vi "Pockels-Modulate funct acq AO seq for mov cor.vi"(7 "Number of POI":i32=3, 11 "Pockels modulation sequence in":dbl[](array[numeric])=array[5601 elements]) -> (1 "Number of blue block insertions":i32, 3 "Pockels modulation sequence out":dbl[](array[numeric]))   [LabVIEW 2020]
uses:
  Typedefs/Imaging Protocols enum.ctl
  Typedefs/Pockels modulation Internal cluster 1.ctl
  Typedefs/Rounding type.ctl
  Global Variables/General Globals.vi
  Globals/gl_Pockels control globals.vi
panel:
  out "Number of ref frame insertions":i32
  out "Case executing":T1(ring)
  in  "Prevent small final chunks (T)":bool
  out "Size of last chunk as % of nominal chunk size":dbl(slide) scale=0.0..100.0
  in  "Enable simulation slider":bool
  out "Output sequence length (ms)":dbl format="%#_g ms"
  out "Points in o/p sequence":i32 format="%.0f points"
  out "Target time between mov.cor. ref triggers (ms)":dbl=2.0 format="%#_g ms"
  out "Ref frame sequence length (ms)":dbl format="%#_g ms"
  out "nominal chunk length (ms)":dbl format="%#_g ms"
  out "Output Sequence Graph":dbl[](graph)
  in  "Ref frame Pockels modulation sequence size":i32(slide)=376 scale=10.0..1200.0
  out "Insertion indexes":i32[](array[numeric])
  out "Length of pockels mod. seq\nduring ROI acquisition (ms)":dbl=198.0 format="%#_g us"
  # "SIMULATION CONTROL"
  # "<--- This is the total length of the retriggerable sequence shown in the graph"
  # "Output Sequence"
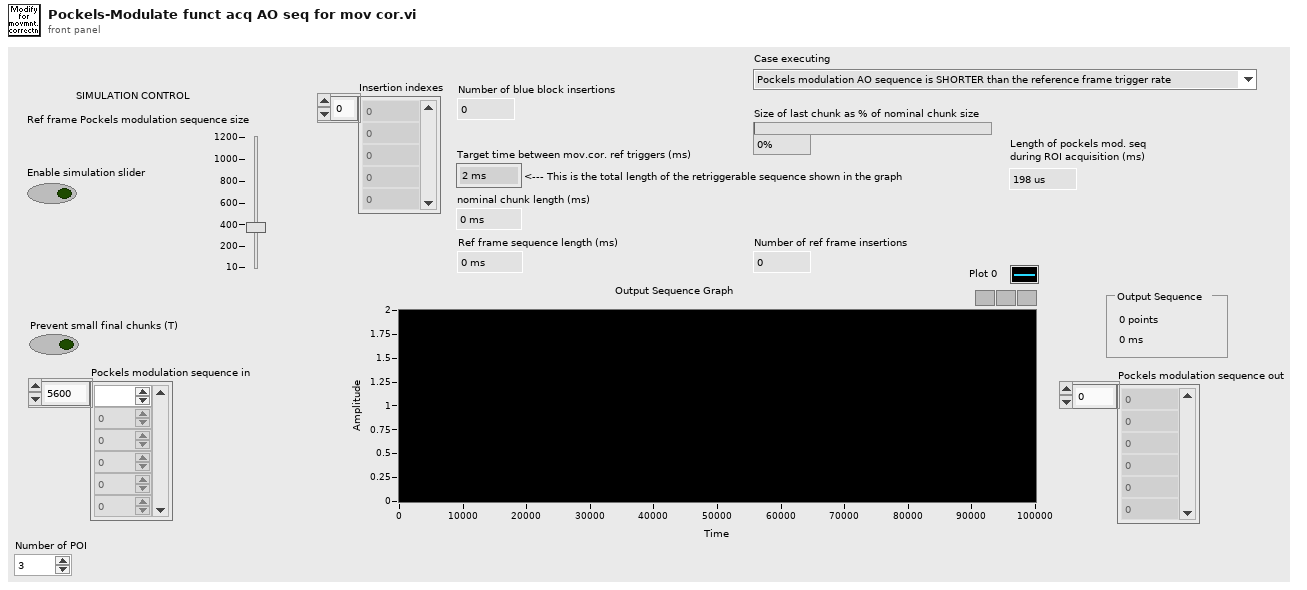
[diagram p1: front panel]
types:
  T1 = enum16{"Pockels modulation AO sequence is SHORTER than the reference frame trigger rate", "Pockels modulation AO sequence is LONGER than the reference frame trigger rate"}
  T2 = typedef "Pockels modulation Internal cluster 1.ctl" = cluster{"Pockels ON \"Pre\" (samples)":i32, "Direction (+-Inf)":T3, "Additional duration to stay ON (samples)":i32, "Not the last ROI":bool}
  T3 = typedef "Rounding type.ctl" = enum16{"No rounding", "Toward +Inf", "Toward -Inf"}
  T4 = typedef "Imaging Protocols enum.ctl" = enum16{"AOL Z-Stack", "Motor Z Stack", "Functional Acquisition", "Single Plane Acquisition", "Volume Acquisition", "Live Imaging", "Live Plane Imaging", "Live Volume Imaging"}
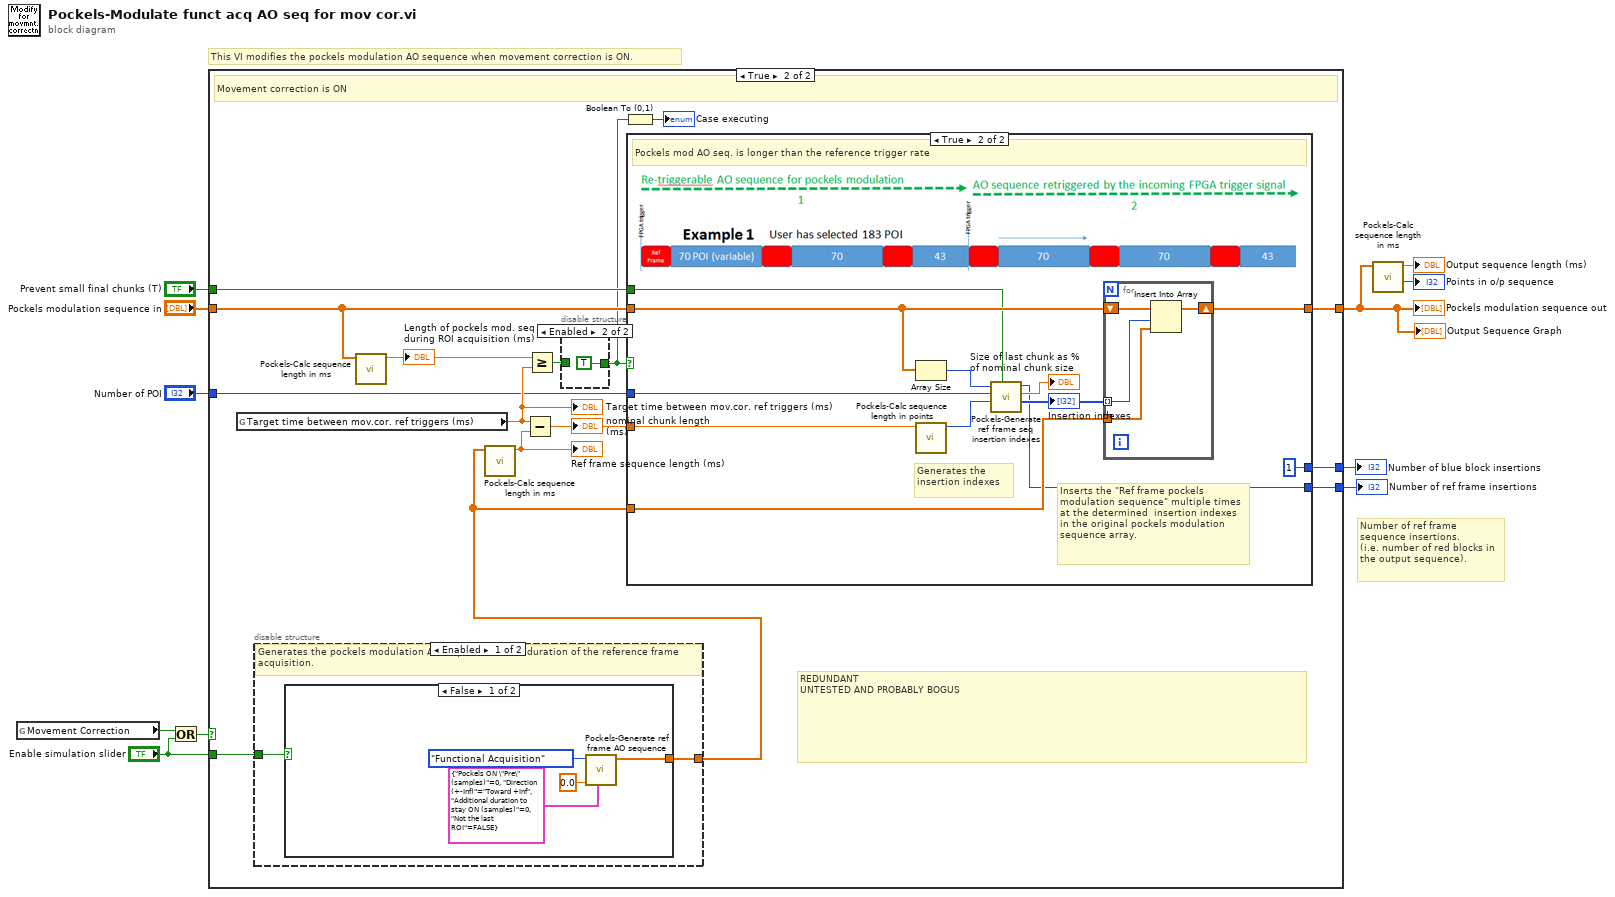
[diagram p0: block diagram]
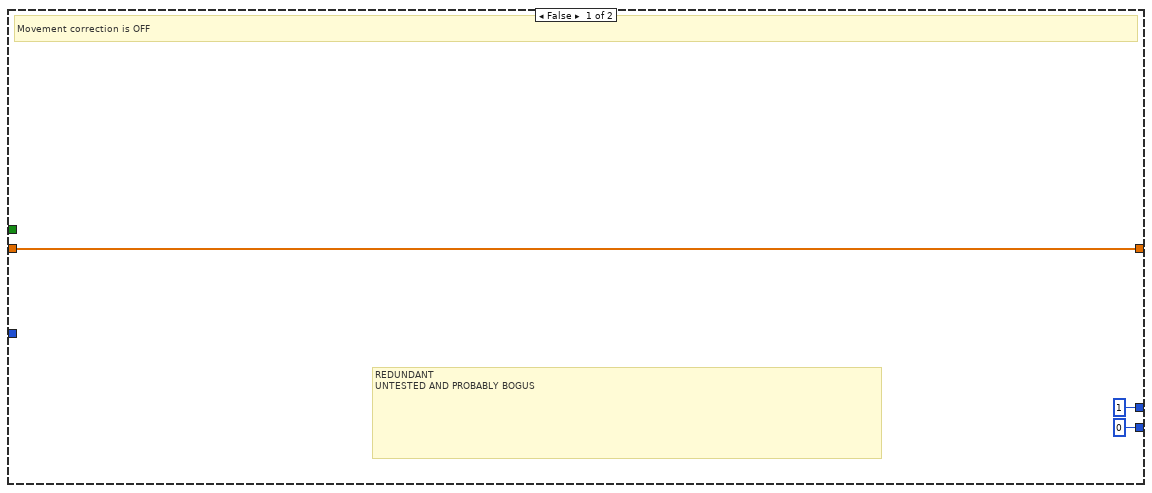
[diagram p2: hidden frame]
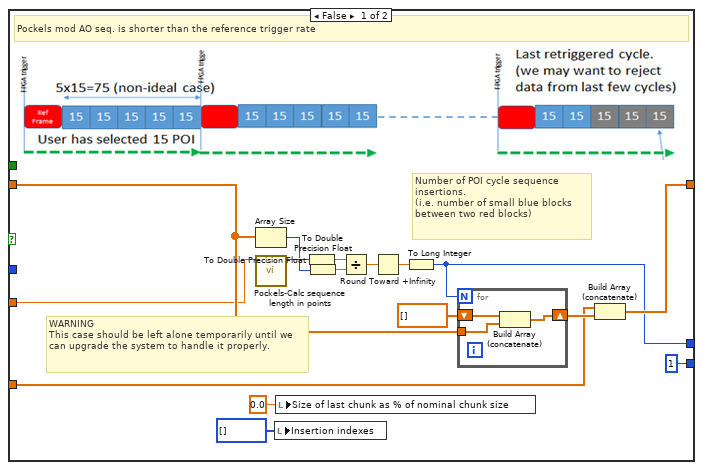
[diagram p4: hidden frame]
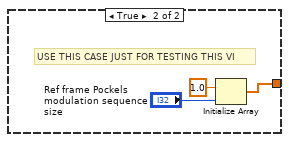
[diagram p5: hidden frame]
diagram:
  # "Number of ref frame sequence insertions.\n(i.e. number of red blocks in the output sequence)."
  # "This VI modifies the pockels modulation AO sequence when movement correction is ON."
  n1 = global read "General Globals.vi" "Movement Correction"() -> (w7:bool)
  n2 = Or(x=w7, y="Enable simulation slider") -> (x .or. y?=w6:bool)
  n3 = case shown="True" w6 {
    tunnel: "Pockels modulation sequence in" -> [w14 w18]
    tunnel: [w14 w28] -> w10
    tunnel: "Enable simulation slider" -> [_ w27]
    tunnel: "Prevent small final chunks (T)" -> [_ w26]
    tunnel: [1 w21] -> w4
    tunnel: [0 ("Number of insertions") w20] -> w3
    tunnel: "Number of POI" -> [_ w17]
    frame False {
      # "REDUNDANT\nUNTESTED AND PROBABLY BOGUS"
      # "Movement correction is OFF"
    }
    frame True {
      # "REDUNDANT\nUNTESTED AND PROBABLY BOGUS"
      # "Movement correction is ON"
      n4 = global read "gl_Pockels control globals.vi" "Target time between mov.cor. ref triggers (ms)"() -> (w22:dbl)
      "Target time between mov.cor. ref triggers (ms)" <- w22
      n5 = disable-structure shown="Enabled" {
        disable-tunnel: [w68 _] -> w19
        disable-tunnel: w27 -> [w67 _]
        frame Enabled {
          # "Generates the pockels modulation AO sequence for the duration of the reference frame acquisition."
          n6 = case shown="False" w67 {
            tunnel: [w72 w73] -> w68
            frame False {
              n7 = call "Pockels-Generate ref frame AO sequence.vi"("Cluster"=T2 {"Pockels ON \"Pre\" (samples)"=0, "Direction (+-Inf)"=enum."Toward +Inf", "Additional duration to stay ON (samples)"=0, "Not the last ROI"=FALSE}, "Previous excess us (us)"=0.0, "Imaging Protocol"=Imaging_Protocols_enum."Functional Acquisition") -> ("Pockels modulation sequence"=w72:dbl[])  [unwired: 4 in, 4 out]
            }
            frame True {
              # "USE THIS CASE JUST FOR TESTING THIS VI"
              n8 = Initialize Array(1.0 ("element"), "Ref frame Pockels modulation sequence size") -> (w73:dbl[])
            }
          }
        }
        frame Disabled {
        }
      }
      n9 = call "Pockels-Calc sequence length in ms.vi"("Pockels modulation sequence in"=w18) -> ("Sequence length (ms)"=w29:dbl)  [unwired: 8 in, 2 out]
      "Length of pockels mod. seq\nduring ROI acquisition (ms)" <- w29
      n10 = call "Pockels-Calc sequence length in ms.vi"("Pockels modulation sequence in"=w19) -> ("Sequence length (ms)"=w25:dbl)  [unwired: 8 in, 2 out]
      "Ref frame sequence length (ms)" <- w25
      n11 = Subtract(x=w22, y=w25) -> (x-y=w24:dbl)
      "nominal chunk length (ms)" <- w24
      n12 = Greater Or Equal?(x=w29, y=w22) -> (x >= y?=w16:bool)
      n13 = disable-structure shown="Enabled" {
        disable-tunnel: [w30 TRUE] -> w15
        disable-tunnel: w16 -> [w30 _]
        frame Disabled {
        }
        frame Enabled {
        }
      }
      n14 = Boolean To (0,1)(Boolean=w15) -> (0, 1=→"Case executing":i16)
      n15 = case shown="True" w15 {
        tunnel: w19 -> [w39 w54]
        tunnel: w18 -> [w38 w60]
        tunnel: [w37 w61] -> w28
        tunnel: w26 -> [_ w56]
        tunnel: w24 -> [w36 w55]
        tunnel: [w33 1] -> w21
        tunnel: [1 ("Number of insertions") w52] -> w20
        tunnel: w17 -> [_ w51]
        frame False {
          # "WARNING\nThis case should be left alone temporarily until we can upgrade the system to handle it properly."
          # "Number of POI cycle sequence insertions.\n(i.e. number of small blue blocks between two red blocks)"
          # "Pockels mod AO seq. is shorter than the reference trigger rate"
          n16 = Array Size(array=w38) -> (size(s)=w45:i32)
          n17 = call "Pockels-Calc sequence length in points.vi"("Sequence length (ms)"=w36) -> ("Points length"=w47:i32)  [unwired: 10 in]
          n18 = local write "Insertion indexes"(i32[] [] ("Insertion indexes")) -> ()
          n19 = local write "Size of last chunk as % of nominal chunk size"(0.0 ("Size of last chunk as % of nominal chunk size")) -> ()
          n20 = To Double Precision Float(number=w47) -> (double precision float=w46:dbl)
          n21 = To Double Precision Float(number=w45) -> (double precision float=w44:dbl)
          n22 = Divide(x=w46, y=w44) -> (x/y=w43:dbl)
          n23 = Round Toward +Infinity(x=w43) -> (ceil(x): smallest int >= x=w42:dbl)
          n24 = To Long Integer(number=w42) -> (32bit integer=w33:i32)
          n25 = for {
            N: w33 -> [_]
            tunnel: w38 -> [w48]
            shift-right: [w49] -> w40
            shift-left: dbl[] [] -> [w50]
            n26 = Build Array (concatenate)(w50, w48) -> (w49:dbl[])
          }
          n27 = Build Array (concatenate)(w39, w40) -> (w37:dbl[])
        }
        frame True {
          # "Generates the insertion indexes"
          # "Inserts the \"Ref frame pockels modulation sequence\" multiple times at the determined  insertion indexes in the original pockels modulation sequence array."
          # "Pockels mod AO seq. is longer than the reference trigger rate"
          n28 = Array Size(array=w60) -> (size(s)=w62:i32)
          n29 = call "Pockels-Calc sequence length in points.vi"("Sequence length (ms)"=w55) -> ("Points length"=w57:i32)  [unwired: 10 in]
          n30 = call "Pockels-Generate ref frame seq insertion indexes.vi"("Prevent small final chunks (T)"=w56, "Nominal chunk length (points)"=w57, "Number of POI"=w51, "Number of points in the original pockels modulation sequence"=w62) -> ("Insertion indexes"=w58:i32[], "Size of last chunk as % of nominal chunk size"=→"Size of last chunk as % of nominal chunk size":dbl, "Number of insertions"=w52:i32)  [unwired: 5 in]
          "Insertion indexes" <- w58
          n31 = for {
            tunnel: w58 -> [w65] mode=indexing
            tunnel: w54 -> [w64]
            shift-right: [w63] -> w61
            shift-left: w60 -> [w66]
            n32 = Insert Into Array(array=w66, index=w65, new element=w64) -> (w63:dbl[])
          }
        }
      }
    }
  }
  "Pockels modulation sequence out" <- w10
  "Output Sequence Graph" <- w10
  "Number of blue block insertions" <- w4
  "Number of ref frame insertions" <- w3
  n33 = call "Pockels-Calc sequence length in ms.vi"("Pockels modulation sequence in"=w10) -> ("Sequence length (points)"=→"Points in o/p sequence":i32, "Sequence length (ms)"=→"Output sequence length (ms)":dbl)  [unwired: 8 in, 1 out]
